vi "add all ciphers.vi"(8 "error in":errorcluster) -> (0 "error out":errorcluster)   [LabVIEW 2016, in "lv tls dll.lvlib"]
uses:
  lv tls dll.lvlib
panel:
  in  "force?":bool
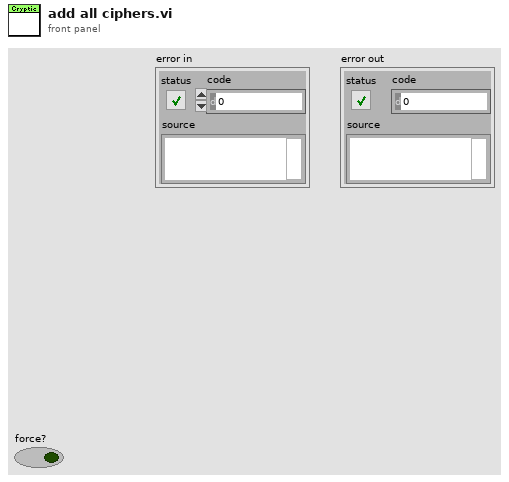
[diagram p1: front panel]
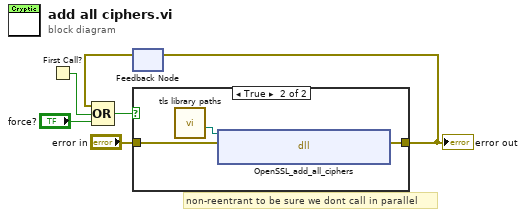
[diagram p0: block diagram]
diagram:
  # "non-reentrant to be sure we dont call in parallel"
  n1 = First Call?() -> (First Call?: T/F=w6:bool)
  n2 = feedback #1() -> (w5:errorcluster)  [unwired: 1 in]
  n3 = Compound Arithmetic op=OR(w5, w6, "force?") -> (w4:bool)
  n4 = case shown="True" w4 {
    tunnel: "error in" -> [w7 w10]
    tunnel: [w7 w8] -> w1
    frame False {
    }
    frame True {
      n5 = call "tls library paths.vi"() -> ("libcrypto"=w9:path)  [unwired: 8 in, 3 out]
      n6 = dll-call lib="C:/Users/IEUser/Desktop/tlssimple/libcrypto-41.dll" fn="OpenSSL_add_all_ciphers"(path in=w9, error in=w10) -> (error out=w8:errorcluster)  [unwired: 2 in, 1 out]
    }
  }
  "error out" <- w1
  n7 = feedback-in #1(w1) -> ()
